vi "Single Control Loop.vi"() -> ()   [LabVIEW 2010]
uses:
  <vilib>/Platform/TimedLoop/XDataNode/XDataNode.xnode
  <vilib>/Platform/TimedLoop/XDataNode/timing_clust.ctl
  <vilib>/Platform/TimedLoop/XDataNode/nitl_modes.ctl
  <vilib>/Platform/TimedLoop/XDataNode/wakeup.ctl
  BotCommands.ctl
  vi/clearpath_interface.lvlib
  <vilib>/Platform/TimedLoop/XDataNode/XDNodeRunTimeDep.lvlib
  <vilib>/NI_Real-Time Target Support.lvlib
panel:
  out "Left":dbl
  out "Right":dbl
  out "Msgs (per sec)":u32
  out "Msgs (total)":u32
  out "Network Timeout?":bool=TRUE
  out "Rotation":dbl(knob) scale=1.0..-1.0
  out "Speed":dbl(knob) scale=-1.0..1.0
  in  "Stop Interface":bool
  in  "Stop Motors?":bool
  in  "stop":bool
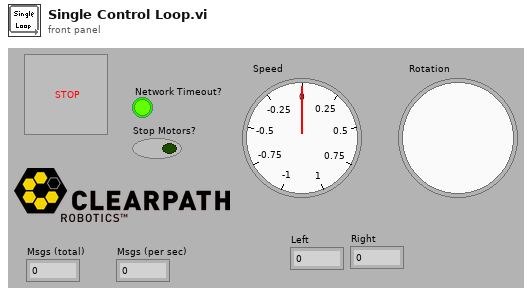
[diagram p1: front panel]
types:
  T1 = cluster{"Xmit Queue":refnum<queue>, "Data Queue":refnum<queue>, "VISA resource name out":refnum<visa-resource-name>, "error out":errorcluster, "Message Data Cluster":cluster{"\nChar Idx":u8, "Num. Char Rem":u8, "Write Index":u8, "Read Index":u8, "Message Data Buffer":u8[][]}}
  T2 = typedef "XDNodeRunTimeDep.lvlib/timing_clust.ctl" = cluster{"Expected End [f-1]":u64, "Actual End [f-1]":u64, "Finished Late? [f-1]":bool, "Expected End [i-1]":u64, "Actual End [i-1]":u64, "Finished Late? [i-1]":bool, "Expected Start [i]":u64, "Actual Start [i]":u64, "Expected Start [f]":u64, "Actual Start [f]":u64, "Source Name":string, "Structure Name":string, "Period":i64, "Deadline":i64, "Offset":i64, "Start":i64, "Priority":i32, "Timeout":i32, "Mode":T3, "Wakeup Reason":T4, "Error":errorcluster, "Source Type":string, "Secondary Source Type":string, "Global End Time":u64, "Global Start Time":u64, "Frame Duration":u64, "Iteration Duration":u64, "Assigned CPU":i32, "I/O Scan Engine Mode":u32}
  T3 = typedef "XDNodeRunTimeDep.lvlib/nitl_modes.ctl" = enum32{"No Change", "Process missed periods, maintain original phase", "Discard missed periods, maintain original phase", "Process missed periods, ignore original phase", "Discard missed periods, ignore original phase"}
  T4 = typedef "XDNodeRunTimeDep.lvlib/wakeup.ctl" = enum32{"Normal", "Aborted", "Asynchronous wakeup", "Timing source error", "Timed loop error", "Timeout"}
  T5 = typedef "BotCommands.ctl" = cluster{"Translational":dbl, "Rotational":dbl}
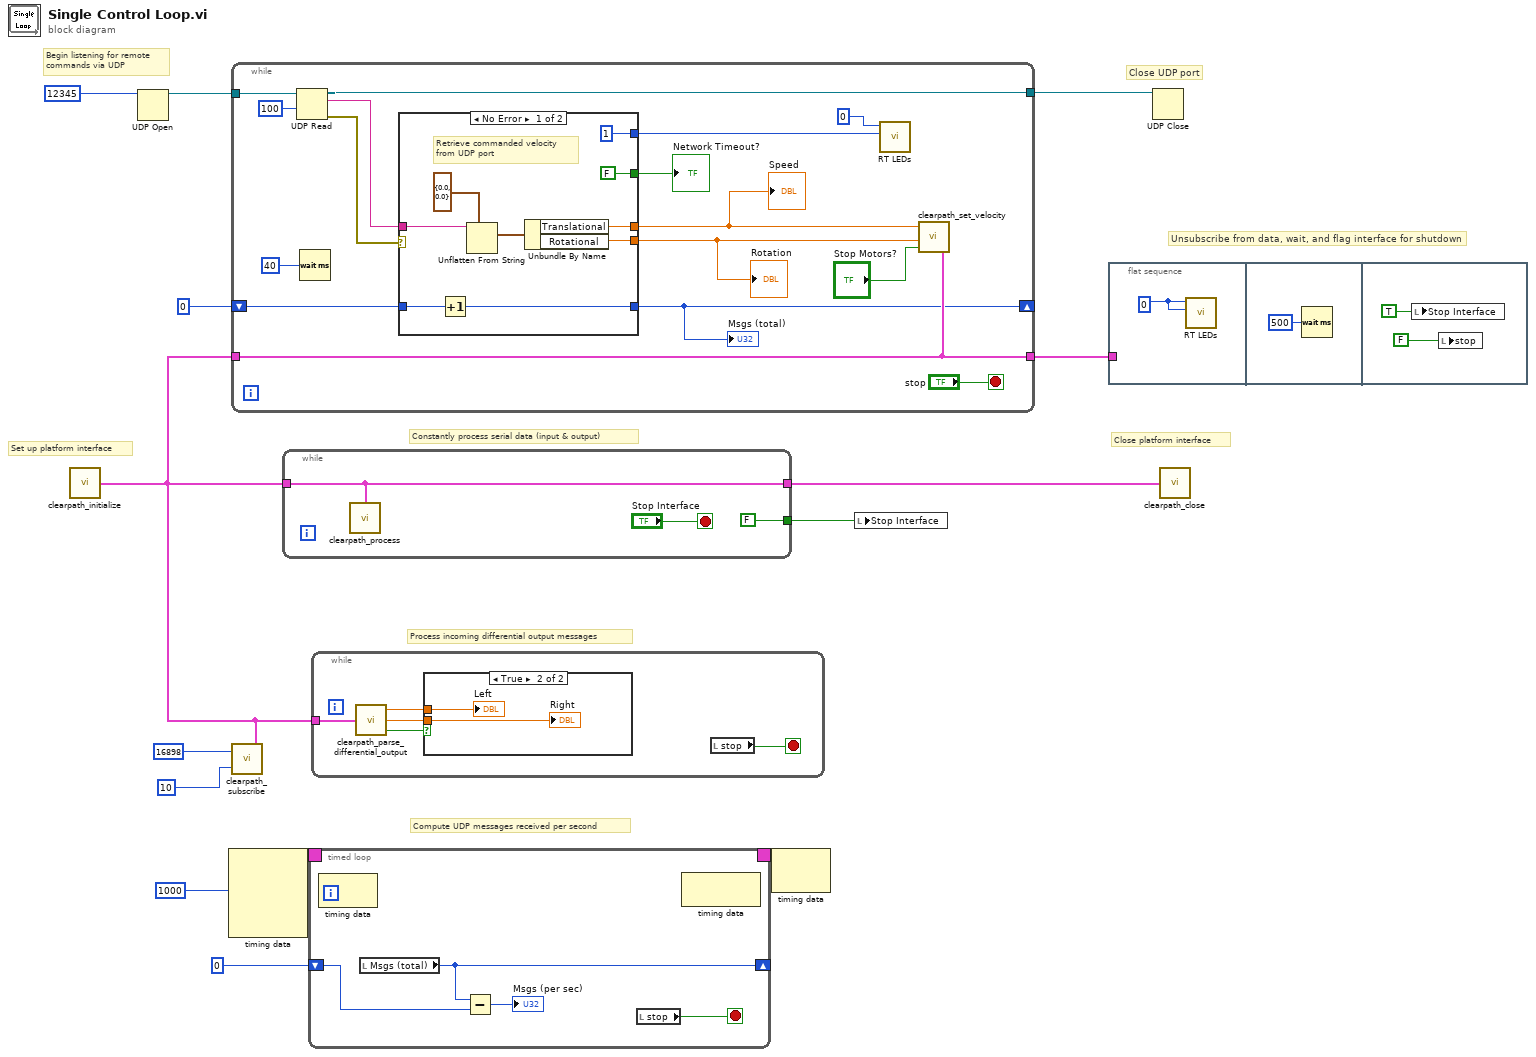
[diagram p0: block diagram]
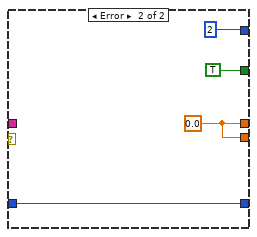
[diagram p3: hidden frame]
diagram:
  # "Compute UDP messages received per second"
  # "Process incoming differential output messages"
  # "Constantly process serial data (input & output)"
  # "Close platform interface"
  # "Close UDP port"
  # "Begin listening for remote\ncommands via UDP"
  # "Unsubscribe from data, wait, and flag interface for shutdown"
  # "Set up platform interface"
  n1 = call "clearpath_initialize.vi"() -> ("ClearpathComm"=w1:T1)  [unwired: 2 in]
  n2 = UDP Open(11:u16 12345 ("port")) -> (port=w13:refnum<k16>)  [unwired: 4 in, 2 out]
  n3 = node-c288(1000) -> (w9:T2)  [unwired: 3 in]
  n4 = while {
    tunnel: w1 -> [w21]
    tunnel: w13 -> [w27]
    tunnel: [w25] -> w14
    tunnel: [w21] -> w11
    shift-right: [w18] -> _
    shift-left: 0 -> [w19]
    stop <- "stop" stop-if-true
    n5 = UDP Read(connection ID=w27, timeout ms (25000)=100) -> (data out=w26:string, error out=w23:errorcluster, 3:w25:refnum<k16>)  [unwired: 2 in, 2 out]
    n6 = Wait (ms)(milliseconds to wait=u32 40) -> ()  [unwired: 1 out]
    n7 = case shown="No Error" w23 {
      tunnel: [w39 w43] -> w29
      tunnel: [w38 w43] -> w28
      tunnel: w26 -> [w35 _]
      tunnel: [FALSE TRUE] -> w22
      tunnel: w19 -> [w33 w41]
      tunnel: [w32 w41] -> w18
      tunnel: [1 2] -> w16
      frame No Error {
        # "Retrieve commanded velocity\nfrom UDP port"
        n8 = Increment(x=w33) -> (x+1=w32:i32)
        n9 = Unflatten From String(type=T5 {"Translational"=0.0, "Rotational"=0.0} ("BotCommands"), binary string=w35) -> (value=w37:T5)  [unwired: 2 in, 3 out]
        n10 = Unbundle By Name(w37) -> ("Translational"=w39:dbl, "Rotational"=w38:dbl)
      }
      frame Error {
        w43 = 0.0 ("Translational")
      }
    }
    "Speed" <- w29
    "Rotation" <- w28
    "Network Timeout?" <- w22
    "Msgs (total)" <- w18
    n11 = call <vilib>:"RT LEDs.vi"("State"=w16, "LED Num"=0) -> ()  [unwired: 4 in, 2 out]
    n12 = call "clearpath_set_velocity.vi"("ClearpathComm"=w21, "Zero Speeds"="Stop Motors?", "Rotational Speed"=w28, "Translational Speed"=w29) -> ()
  }
  n13 = call "clearpath_subscribe.vi"("ClearpathComm"=w1, "Frequency"=10, "Message Type"=16898) -> ()
  n14 = while {
    tunnel: w1 -> [w44]
    tunnel: [w44] -> w5
    tunnel: [FALSE ("Stop Interface")] -> w4
    stop <- "Stop Interface" stop-if-true
    n15 = call "clearpath_process.vi"("ClearpathComm"=w44) -> ()
  }
  n16 = timed-loop {
    timing: w9 -> [_]
    timing-out: [_] -> w8
    shift-right: [w49] -> _
    shift-left: 0 -> [w50]
    stop <- w47 stop-if-true
    n17 = node-c288() -> ()  [unwired: 1 in, 1 out]
    n18 = local read "Msgs (total)"() -> (w49:u32)
    n19 = Subtract(x=w49, y=w50) -> (x-y=→"Msgs (per sec)":u32)
    n20 = local read "stop"() -> (w47:bool)
    n21 = node-c288() -> ()  [unwired: 1 in, 1 out]
  }
  n22 = while {
    tunnel: w1 -> [w54]
    stop <- w53 stop-if-true
    n23 = call "clearpath_parse_differential_output.vi"("ClearpathComm"=w54) -> ("Data Valid?"=w55:bool, "Right Output"=w56:dbl, "Left Output"=w57:dbl)
    n24 = case shown="True" w55 {
      tunnel: w57 -> [_ w59]
      tunnel: w56 -> [_ w58]
      frame False {
      }
      frame True {
        "Left" <- w59
        "Right" <- w58
      }
    }
    n25 = local read "stop"() -> (w53:bool)
  }
  n26 = node-c288(w8) -> ()  [unwired: 1 out]
  n27 = local write "Stop Interface"(w4) -> ()
  n28 = flat-sequence {
    tunnel: w11 -> [_]
    frame #0 {
      w60 = 0
      n29 = call <vilib>:"RT LEDs.vi"("State"=w60, "LED Num"=w60) -> ()  [unwired: 4 in, 2 out]
    }
    frame #1 {
      n30 = Wait (ms)(milliseconds to wait=u32 500) -> ()  [unwired: 1 out]
    }
    frame #2 {
      n31 = local write "Stop Interface"(TRUE ("Stop Interface")) -> ()
      n32 = local write "stop"(FALSE ("stop")) -> ()
    }
  }
  n33 = UDP Close(connection ID=w14) -> ()  [unwired: 1 in, 2 out]
  n34 = call "clearpath_close.vi"("ClearpathComm"=w5) -> ()
